vi "Set Send Icon.vi"(8 "error in (no error)":errorcluster, 9 "Icon in":refnum<class "Icon.lvclass">, 10 "Send Method path":path, 11 "AppInst":refnum<vi>) -> (0 "error out":errorcluster, 1 "Icon out":refnum<class "Icon.lvclass">)   [LabVIEW 2020, in "Message Maker.lvlib"]
uses:
  Message Maker.lvlib
  <vilib>/LabVIEW Icon API/LabVIEW Icon API.lvlib
  <vilib>/picture/picture.llb/imagedata.ctl
  <vilib>/Utility/miscctls.llb/LVPoint32TypeDef.ctl
  Localized Strings.vi
  <vilib>/LabVIEW Icon API/API_User Layer Data.ctl
  <vilib>/LabVIEW Icon API/lv_icon/Classes/Icon/Icon.lvclass
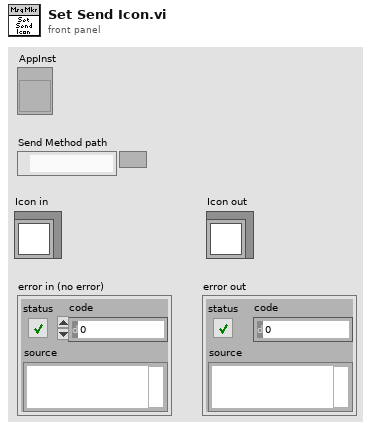
[diagram p1: front panel]
types:
  T1 = typedef "LabVIEW Icon API.lvlib/API_User Layer Data.ctl" = cluster{"Layer name":string, "Origin":T2, "Icon image data":T3}
  T2 = typedef "LVPoint32TypeDef.ctl" = cluster{"Horizontal":i32, "Vertical":i32}
  T3 = typedef "imagedata.ctl" = cluster{"image type":i32, "image depth":i32, "image":u8[], "mask":u8[], "colors":u32[], "Rectangle":cluster{"left":i16, "top":i16, "right":i16, "bottom":i16}}
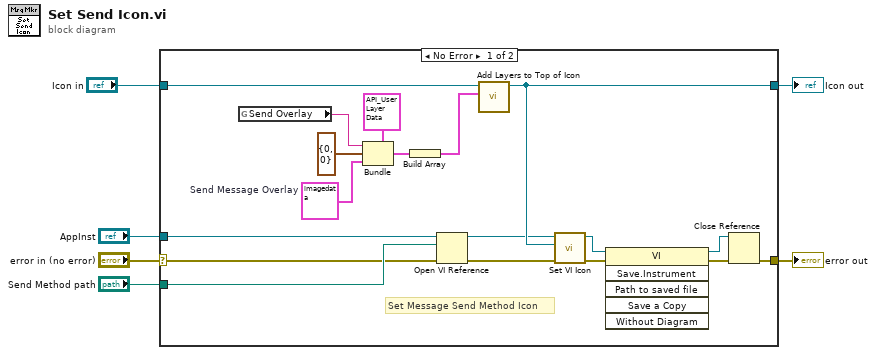
[diagram p0: block diagram]
diagram:
  n1 = case shown="No Error" "error in (no error)" {
    selector: "error in (no error)" -> [w10 w25]
    tunnel: "AppInst" -> [w24 _]
    tunnel: [w23 w25] -> w5
    tunnel: "Send Method path" -> [w20 _]
    tunnel: "Icon in" -> [w19 w26]
    tunnel: [w15 w26] -> w2
    frame No Error {
      w17 = T3 {"image type"=0, "image depth"=24, "image"=array[3072 elements], "mask"=[0, 0, 0, 0, 0, 0, 0, 0, 0, 0, 0, 0, 0, 0, 0, 0, 0, 0, 0, 0, 0, 0, 0, 0, 0, 0, 0, 0, 0, 0, 0, 0, 0, 0, 0, 0, 0, 0, 0, 0, 0, 0, 0, 0, 0, 0, 0, 0, 0, 0, 0, 0, 0, 0, 0, 0, 0, 0, 0, 0, 0, 0, 0, 0, 0, 0, 0, 0, 0, 0, 0, 0, 0, 0, 0, 0, 0, 0, 0, 0, 0, 0, 0, 0, 0, 0, 0, 112, 0, 0, 1, 252, 0, 0, 3, 254, 0, 0, 3, 254, 0, 0, 7, 255, 0, 0, 7, 255, 0, 0, 7, 255, 0, 0, 3, 254, 0, 0, 3, 254, 0, 0, 1, 252, 0, 0, 0, 112], "colors"=[], "Rectangle"={"left"=0, "top"=0, "right"=32, "bottom"=32}}  # Send Message Overlay
      # "Set Message Send Method Icon"
      n2 = global read "Localized Strings.vi" "Send Overlay"() -> (w13:string)
      n3 = Bundle(cluster=T1 {"Layer name"="", "Origin"={"Horizontal"=0, "Vertical"=0}, "Icon image data"={"image type"=0, "image depth"=0, "image"=[], "mask"=[], "colors"=[], "Rectangle"={"left"=0, "top"=0, "right"=0, "bottom"=0}}} ("User layer"), "Layer name"=w13, "Origin"=T2 {"Horizontal"=0, "Vertical"=0}, "Icon image data"=w17) -> (w16:T1)
      n4 = Build Array(w16) -> (w12:T1[])
      n5 = Open VI Reference(application reference (local)=w24, vi path=w20, error in (no error)=w10) -> (vi reference=w14:refnum<vi>, error out=w21:errorcluster)  [unwired: 3 in]
      n6 = call "Add Layers to Top of Icon.vi"("User layers"=w12, "Icon.lvclass in"=w19) -> ("Icon.lvclass out"=w15:refnum<class "Icon.lvclass">)  [unwired: 9 in]
      n7 = call <vilib>:"Set VI Icon.vi"("error in (no error)"=w21, "Icon"=w15, "VI Refnum in"=w14) -> ("error out"=w22:errorcluster, "VI Refnum out"=w8:refnum<vi>)  [unwired: 7 in]
      n8 = invoke class="VI" method="Save.Instrument"(reference=w8, error in=w22) -> (reference out=w7:refnum<vi>, error out=w9:errorcluster)  [unwired: 4 in, 4 out]
      n9 = Close Reference(reference=w7, error in (no error)=w9) -> (error out=w23:errorcluster)
    }
    frame Error {
    }
  }
  "error out" <- w5
  "Icon out" <- w2
